vi "Create From Template.vi"() -> ()   [LabVIEW 2021]
uses:
  _Create From Template/Script Strategy/Script Strategy/Script Strategy.lvclass
  _Create From Template/_Create From Template.lvlib
  _Create From Template/Script Strategy/Script Strategy.lvlib
panel:
  in  "Template":string(combo)
  in  "Name":string
  in  "Create":bool
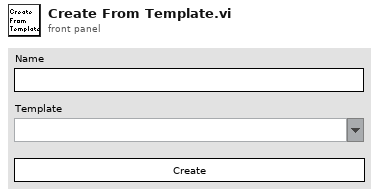
[diagram p1: front panel]
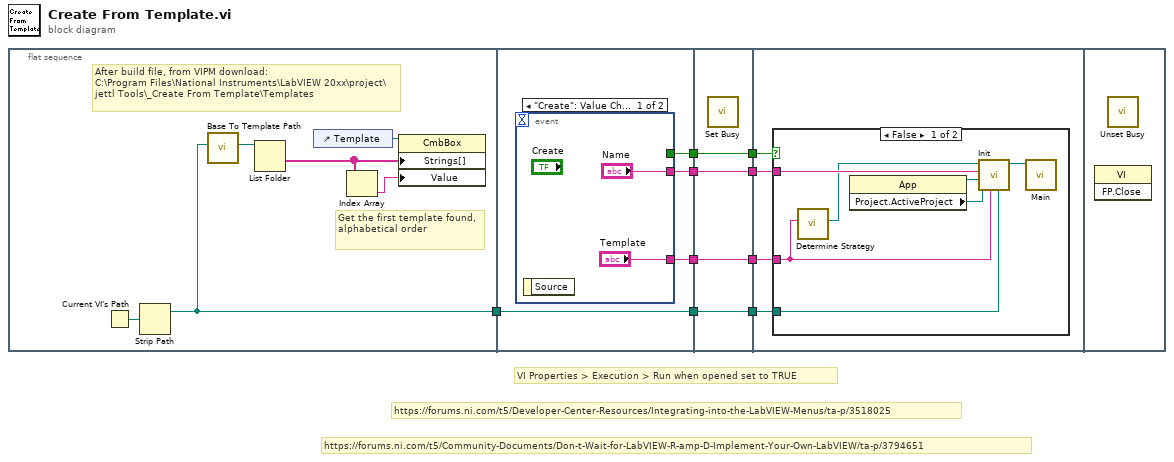
[diagram p0: block diagram]
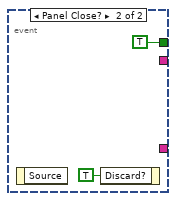
[diagram p2: hidden frame]
diagram:
  # "https://forums.ni.com/t5/Community-Documents/Don-t-Wait-for-LabVIEW-R-amp-D-Implement-Your-Own-LabVIEW/ta-p/3794651"
  # "https://forums.ni.com/t5/Developer-Center-Resources/Integrating-into-the-LabVIEW-Menus/ta-p/3518025"
  # "VI Properties > Execution > Run when opened set to TRUE"
  n1 = flat-sequence {
    tunnel: [w10] -> w9
    tunnel: w9 -> [w19]
    tunnel: [w19] -> w8
    tunnel: [w18] -> w6
    tunnel: [w17] -> w4
    tunnel: [w16] -> w2
    tunnel: w8 -> [w27]
    tunnel: [w27] -> w7
    tunnel: w6 -> [w26]
    tunnel: [w26] -> w5
    tunnel: w4 -> [w25]
    tunnel: [w25] -> w3
    tunnel: w2 -> [w24]
    tunnel: [w24] -> w1
    tunnel: w7 -> [w31]
    tunnel: w5 -> [w30]
    tunnel: w3 -> [w29]
    tunnel: w1 -> [w28]
    frame #0 {
      # "After build file, from VIPM download:\nC:\\Program Files\\National Instruments\\LabVIEW 20xx\\project\\jettl Tools\\_Create From Template\\Templates"
      # "Get the first template found, alphabetical order"
      n2 = Current VI's Path() -> (path=w13:path)
      n3 = Strip Path(path=w13) -> (stripped path=w10:path)  [unwired: 1 out]
      n4 = call "Base To Template Path.vi"("Base Path"=w10) -> ("Templates Path"=w12:path)  [unwired: 10 in]
      n5 = List Folder(path=w12) -> (folder names=w11:string[])  [unwired: 3 in, 3 out]
      n6 = control-ref of="Template"() -> (w14:refnum<vi>)
      n7 = Index Array(array=w11) -> (element=w15:string)  [unwired: 1 in]
      n8 = property class="CmbBox"(reference=w14, "Strings[]"=w11, "Value"=w15) -> ()  [unwired: 1 in, 2 out]
    }
    frame #1 {
      n9 = event shown="[0] \"Create\": Value Change" {
        selector: _ -> [_ _]
        dyn-events: _ -> [_ _]
        timeout: _ -> [_ _]
        tunnel: ["Name" _] -> w18
        tunnel: [_ TRUE] -> w17
        tunnel: ["Template" _] -> w16
        event "Create": Value Change {
          n10 = event-data() -> ()  [unwired: 1 in, 1 out]
        }
        event Panel Close? {
          n11 = event-data() -> ()  [unwired: 1 in, 1 out]
          n12 = event-data("Discard?"=TRUE) -> ()  [unwired: 1 in, 1 out]
        }
      }
    }
    frame #2 {
      n13 = call <vilib>:"Set Busy.vi"() -> ()  [unwired: 10 in, 2 out]
    }
    frame #3 {
      n14 = case shown="False" w29 {
        tunnel: w30 -> [w38 _]
        tunnel: w28 -> [w33 _]
        tunnel: w31 -> [w32 _]
        frame False {
          n15 = call "Determine Strategy.vi"("Template"=w33) -> ("Script Strategy"=w35:refnum<class "Script Strategy.lvclass">)  [unwired: 10 in]
          n16 = property class="App"() -> (reference out=w37:refnum<vi>, "Project.ActiveProject"=w36:refnum<vi>)  [unwired: 2 in, 1 out]
          n17 = call-dynamic "Init.vi"("Base Path"=w32, "Template Name"=w33, "Project:Active Project"=w36, "Application Instance"=w37, "Name"=w38, "Script Strategy in"=w35) -> ("Script Strategy out"=w34:refnum<class "Script Strategy.lvclass">)  [unwired: 5 in]
          n18 = call-dynamic "Main.vi"("Script Strategy in"=w34) -> ()  [unwired: 11 in]
        }
        frame True {
        }
      }
    }
    frame #4 {
      n19 = invoke class="VI" method="FP.Close"() -> ()  [unwired: 3 in, 3 out]
      n20 = call <vilib>:"Unset Busy.vi"() -> ()  [unwired: 11 in, 1 out]
    }
  }
